vi "Read Helm Status Message.vi"(8 "error in (no error)":errorcluster, 11 "Helm Status Message in":refnum<class "Helm Status Message.lvclass">) -> (0 "error out":errorcluster, 2 "Helm Status":T1 {"Gains"."D (Td)" format="%#_9f"; "Gains"."I (Ti)" format="%#_9f"; "Gains"."P (Kc)" format="%#.9f"}, 3 "Helm Status Message out":refnum<class "Helm Status Message.lvclass">)   [LabVIEW 2015, in "RDS Child Messages.lvlib" / "Helm Status Message.lvclass"]
uses:
  Helm Status Message.lvclass
  Helm Status Control.ctl
  Actors/RDS Helm Actor/RDS Helm Actor/Helm State.ctl
  Heading Command/Heading Command Cntrl.ctl
  Steering Command/Steering Command Cntrl.ctl
  PID Gains/PID Gains Control.ctl
  Helm Status Message.lvclass/Helm Status Message.ctl
  Actors/RDS Helm Actor/RDS Helm Actor.lvlib
  RDS Child Messages.lvlib
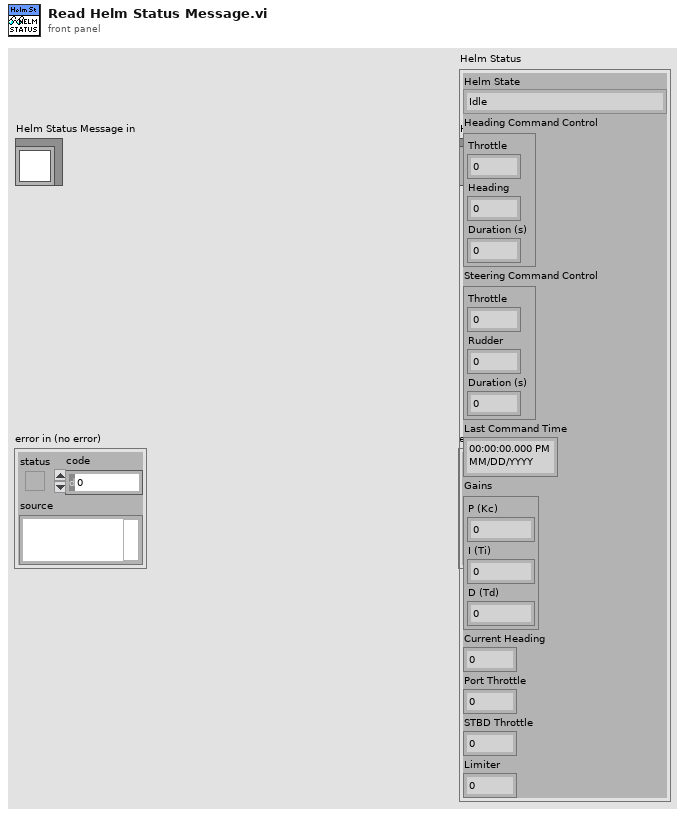
[diagram p1: front panel]
types:
  T1 = typedef "RDS Child Messages.lvlib/Helm Status Control.ctl" = cluster{"Helm State":T2, "Heading Command Control":T3, "Steering Command Control":T4, "Last Command Time":timestamp, "Gains":T5, "Current Heading":dbl, "Port Throttle":i16, "STBD Throttle":i16, "Limiter":dbl}
  T2 = typedef "RDS Helm Actor.lvlib/Helm State.ctl" = enum16{"Idle", "Executing Heading Command", "Executing Steering Command"}
  T3 = typedef "RDS Child Messages.lvlib/Heading Command Cntrl.ctl" = cluster{"Throttle":i16, "Heading":sgl, "Duration (s)":i16}
  T4 = typedef "RDS Child Messages.lvlib/Steering Command Cntrl.ctl" = cluster{"Throttle":i16, "Rudder":i8, "Duration (s)":u16}
  T5 = typedef "RDS Child Messages.lvlib/PID Gains Control.ctl" = cluster{"P (Kc)":sgl, "I (Ti)":sgl, "D (Td)":sgl}
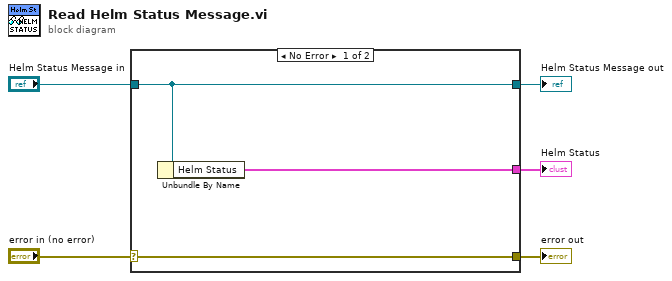
[diagram p0: block diagram]
diagram:
  n1 = case shown="No Error" "error in (no error)" {
    selector: "error in (no error)" -> [w8 w9]
    tunnel: [w8 w9] -> w4
    tunnel: [w7 w10] -> w2
    tunnel: "Helm Status Message in" -> [w7 w10]
    tunnel: [w6 _] -> w1
    frame No Error {
      n2 = Unbundle By Name(w7) -> ("Helm Status"=w6:T1)
    }
    frame Error {
    }
  }
  "error out" <- w4
  "Helm Status Message out" <- w2
  "Helm Status" <- w1
